vi "DDS RAM Set.vi"(8 "error in (no error)":errorcluster, 11 "DDS Box Cluster":T1 {"Array of DDS Channels (4)"."Channel Parameters"."Ref Clock Rate [kHz]" min=0.0}) -> (0 "error out":errorcluster, 3 "DDS box device reference":T2={"NI USB-8451 device reference"="", "DIO port"=0, "Serial Clock Rate [kHz]"=1000})   [LabVIEW 2013]
uses:
  DDS_box_device_reference.ctl
  <vilib>/ni845x/ni845x.llb/ni845xControl.ctl
  DDS_box_cluster.ctl
  array_of_DDS_channels.ctl
  DDS_channel.ctl
  array_of_DDS_profiles.ctl
  DDS_profile.ctl
  DDS RAM mode.ctl
  AD9910 registers.ctl
  <vilib>/gmath/NI_Gmath.lvlib
  cesium_controller/DDS/DDS.lvclass
panel:
  out "RAM data":u8[][](array[numeric])
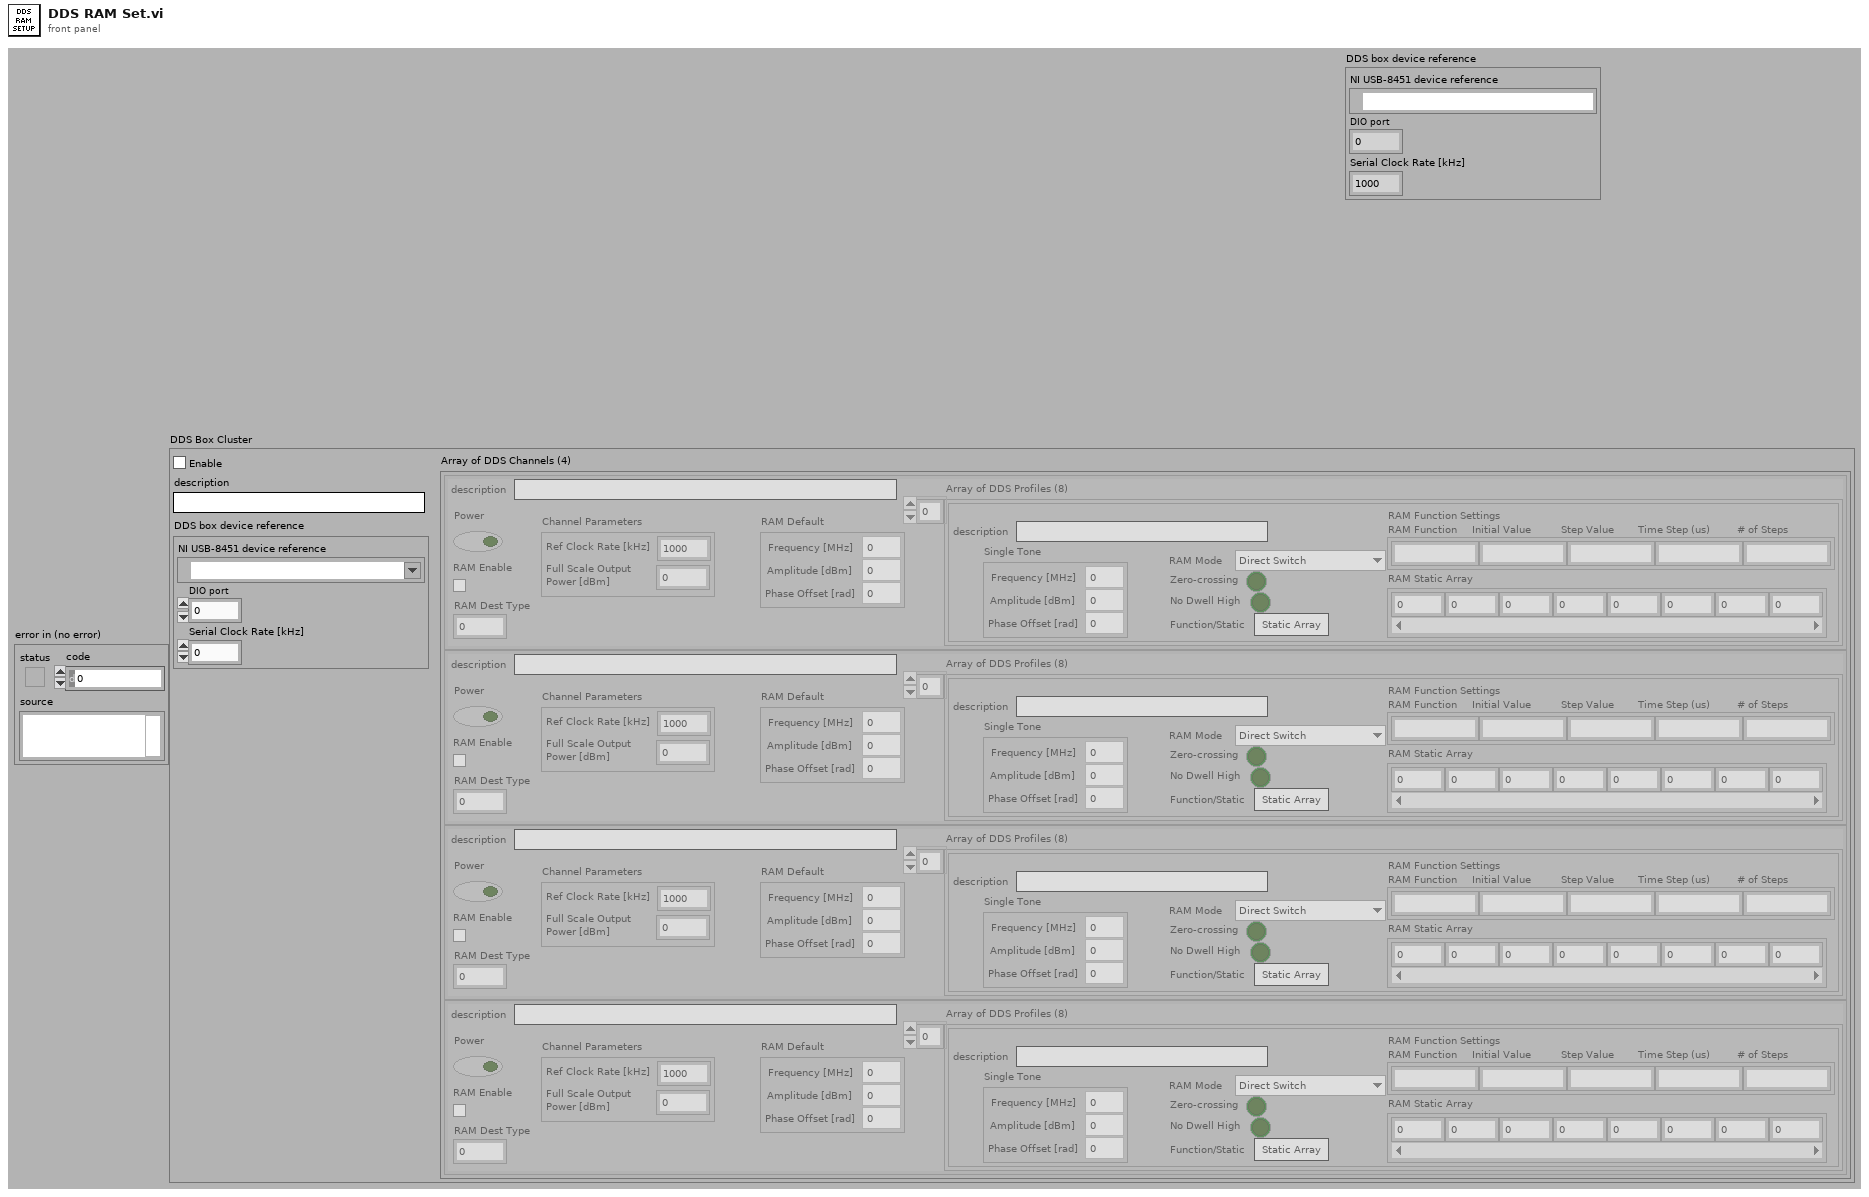
[diagram p1: front panel]
types:
  T1 = typedef "DDS_box_cluster.ctl" = cluster{"DDS box device reference":T2, "Array of DDS Channels (4)":T4, "Enable":bool, "description":string}
  T2 = typedef "DDS_box_device_reference.ctl" = cluster{"NI USB-8451 device reference":T3, "DIO port":u8, "Serial Clock Rate [kHz]":u16}
  T3 = typedef "ni845xControl.ctl" = refnum<k21>
  T4 = typedef "DDS.lvclass/array_of_DDS_channels.ctl" = T5[]
  T5 = typedef "DDS.lvclass/DDS_channel.ctl" = cluster{"Power":bool, "Channel Parameters":cluster{"Ref Clock Rate [kHz]":dbl, "Full Scale Output\nPower [dBm]":dbl}, "RAM Enable":bool, "RAM Dest Type":u8, "RAM Default":cluster{"Frequency [MHz]":dbl, "Amplitude [dBm]":dbl, "Phase Offset [rad]":dbl}, "Array of DDS Profiles (8)":T6, "description":string}
  T6 = typedef "DDS.lvclass/array_of_DDS_profiles.ctl" = T7[]
  T7 = typedef "DDS_profile.ctl" = cluster{"Single Tone":cluster{"Frequency [MHz]":dbl, "Amplitude [dBm]":dbl, "Phase Offset [rad]":dbl}, "RAM Mode ":T8, "Zero-crossing":bool, "No Dwell High":bool, "Function/Static":bool, "RAM Function Settings":string[], "RAM Static Array":dbl[], "description":string}
  T8 = typedef "DDS RAM mode.ctl" = enum16{"Direct Switch", "Ramp Up", "Bidirectional Ramp", "Continuous Bidirectional Ramp", "Continuous Recirculate", "Direct Switch 2", "Direct Switch 3", "Direct Switch 4"}
  T9 = typedef "AD9910 registers.ctl" = enum16{"CFR1", "CFR2", "CFR3", "Auxiliary DAC Control", "I/0 Update Rate", "Frequency Tuning Word", "Phase Offset Word", "Amplitude Scale Factor", "Multichip Sync", "Digital Ramp Limit", "Digital Ramp Step Size", "Digital Ramp Rate", "Single Tone Profile 0", "Single Tone Profile 1", "Single Tone Profile 2", "Single Tone Profile 3", "Single Tone Profile 4", "Single Tone Profile 5", "Single Tone Profile 6", "Single Tone Profile 7", "RAM Profile 0", "RAM Profile 1", "RAM Profile 2", "RAM Profile 3", "RAM Profile 4", "RAM Profile 5", "RAM Profile 6", "RAM Profile 7", "RAM"}
  T10 = cluster{"Ref Clock Rate [kHz]":dbl, "Full Scale Output\nPower [dBm]":dbl}
  T11 = cluster{"Frequency [MHz]":dbl, "Amplitude [dBm]":dbl, "Phase Offset [rad]":dbl}
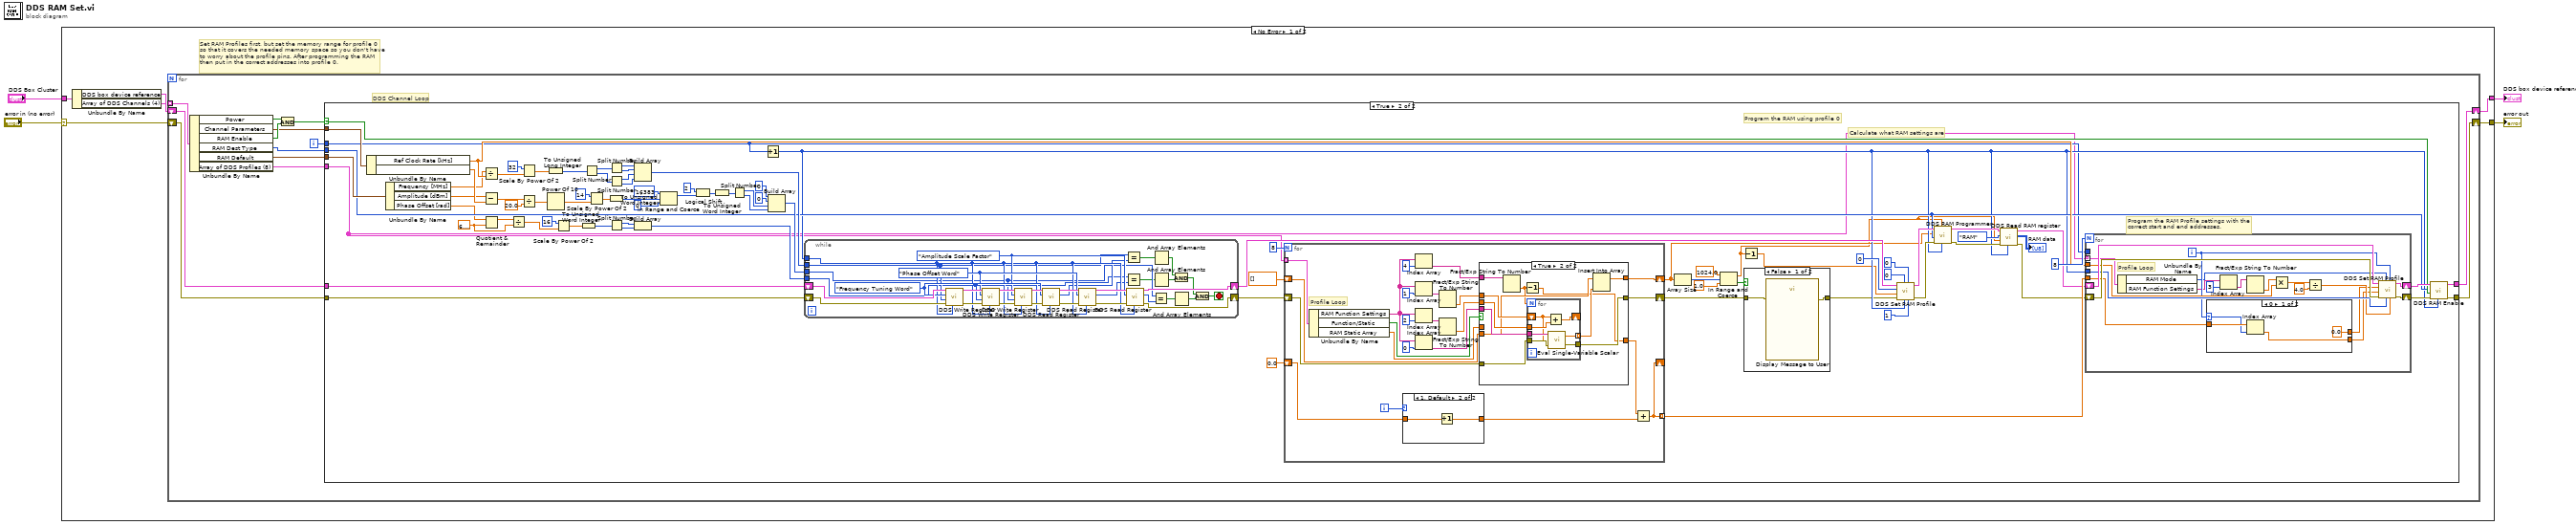
[diagram p0: block diagram]
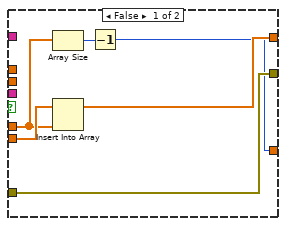
[diagram p5: hidden frame]
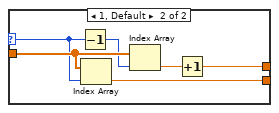
[diagram p6: hidden frame]
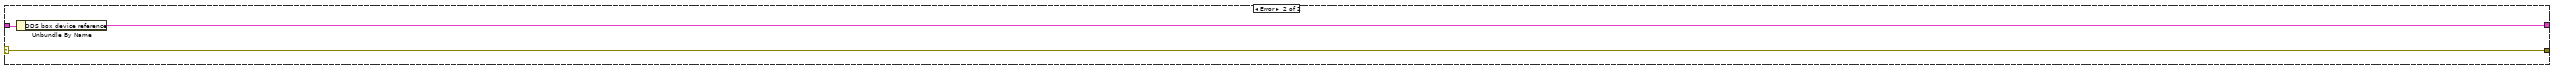
[diagram p7: hidden frame]
diagram:
  n1 = case shown="No Error" "error in (no error)" {
    selector: "error in (no error)" -> [w6 w225]
    tunnel: [w10 w226] -> w4
    tunnel: [w9 w225] -> w3
    tunnel: "DDS Box Cluster" -> [w5 w224]
    frame No Error {
      # "Set RAM Profiles first, but set the memory range for profile 0\nso that it covers the needed memory space so you don't have\nto worry about the profile pins. After programming the RAM\nthen put in the correct addresses into profile 0."
      n2 = Unbundle By Name(w5) -> ("DDS box device reference"=w8:T2, "Array of DDS Channels (4)"=w7:T4)
      n3 = for {
        shift-right: [w23] -> w10
        shift-left: w8 -> [w21]
        shift-right: [w22] -> w9
        shift-left: w6 -> [w20]
        tunnel: w7 -> [w18] mode=indexing
        i -> [w19]
        # "DDS Channel Loop"
        n4 = Unbundle By Name(w18) -> ("Power"=w17:bool, "Channel Parameters"=w14:T10, "RAM Enable"=w16:bool, "RAM Dest Type"=w13:u8, "RAM Default"=w12:T11, "Array of DDS Profiles (8)"=w11:T6)
        n5 = And(x=w17, y=w16) -> (x .and. y?=w15:bool)
        n6 = case shown="True" w15 {
          selector: w15 -> [_ w56]
          tunnel: w12 -> [_ w81]
          tunnel: w14 -> [_ w80]
          tunnel: [w25 w59] -> w23
          tunnel: [w24 w57] -> w22
          tunnel: w21 -> [w25 w61]
          tunnel: w20 -> [w24 w26]
          tunnel: w13 -> [_ w55]
          tunnel: w19 -> [_ w31]
          tunnel: w11 -> [_ w30]
          frame False {
          }
          frame True {
            w95 = 6.283185307179586
            # "Program the RAM Profile settings with the\ncorrect start and end addresses."
            # "Program the RAM using profile 0"
            # "Calculate what RAM settings are"
            n7 = Unbundle By Name(w80) -> ("Ref Clock Rate [kHz]"=w74:dbl, "Full Scale Output\nPower [dBm]"=w79:dbl)
            n8 = Unbundle By Name(w81) -> ("Frequency [MHz]"=w29:dbl, "Amplitude [dBm]"=w28:dbl, "Phase Offset [rad]"=w27:dbl)
            n9 = Divide(x=w29, y=w74) -> (x/y=w109:dbl)
            n10 = Subtract(x=w28, y=w79) -> (x-y=w91:dbl)
            n11 = Quotient & Remainder(x=w27, y=w95) -> (x-y*floor(x/y)=w98:dbl)  [unwired: 1 out]
            n12 = Divide(x=w98, y=w95) -> (x/y=w96:dbl)
            n13 = Scale By Power Of 2(n=32 ("x"), x=w109) -> (x*2^n=w107:dbl)
            n14 = Divide(x=w91, y=20.0) -> (x/y=w89:dbl)
            n15 = To Unsigned Long Integer(number=w107) -> (unsigned 32bit integer=w104:u32)
            n16 = Power Of 10(x=w89) -> (10^x=w88:dbl)
            n17 = Scale By Power Of 2(n=16, x=w96) -> (x*2^n=w97:dbl)
            n18 = To Unsigned Word Integer(number=w97) -> (unsigned 16bit integer=w94:u16)
            n19 = Split Number(x=w104) -> (hi(x)=w105:u16, lo(x)=w106:u16)
            n20 = Scale By Power Of 2(n=14, x=w88) -> (x*2^n=w86:dbl)
            n21 = To Unsigned Word Integer(number=w86) -> (unsigned 16bit integer=w51:u16)
            n22 = Split Number(x=w105) -> (hi(x)=w103:u8, lo(x)=w102:u8)
            n23 = Split Number(x=w106) -> (hi(x)=w101:u8, lo(x)=w100:u8)
            n24 = Split Number(x=w94) -> (hi(x)=w93:u8, lo(x)=w92:u8)
            n25 = Build Array(w103, w102, w101, w100) -> (w78:u8[])
            n26 = Build Array(w93, w92) -> (w76:u8[])
            n27 = In Range and Coerce(upper limit=u32 16383, x=w51, lower limit=u32 0) -> (coerced(x)=w50:u32)  [unwired: 1 out]
            n28 = Logical Shift(y=i8 2, x=w50) -> (x << y=w49:u32)
            n29 = To Unsigned Word Integer(number=w49) -> (unsigned 16bit integer=w48:u16)
            n30 = Split Number(x=w48) -> (hi(x)=w84:u8, lo(x)=w85:u8)
            n31 = Increment(x=w31) -> (x+1=w42:i32)
            n32 = Build Array(u8 0 ("element"), u8 0 ("element"), w84, w85) -> (w77:u8[])
            n33 = while {
              tunnel: w78 -> [w125]
              tunnel: w77 -> [w123]
              tunnel: w76 -> [w124]
              tunnel: w42 -> [w127]
              shift-right: [w131] -> w73
              shift-left: w61 -> [w140]
              shift-right: [w132] -> w71
              shift-left: w26 -> [w139]
              stop <- w113 stop-if-true
              w128 = AD9910_registers."Amplitude Scale Factor" ("Register")
              w129 = AD9910_registers."Phase Offset Word" ("Register")
              w130 = AD9910_registers."Frequency Tuning Word" ("Register")
              n34 = call "DDS Write Register.vi"("channel number (1)"=w127, "error in (no error)"=w139, "Write Data"=w125, "Register"=w130, "DDS ref in"=w140) -> ("error out"=w143:errorcluster, "DDS ref out"=w144:T2)  [unwired: 5 in]
              n35 = call "DDS Write Register.vi"("channel number (1)"=w127, "error in (no error)"=w143, "Write Data"=w124, "Register"=w129, "DDS ref in"=w144) -> ("error out"=w141:errorcluster, "DDS ref out"=w142:T2)  [unwired: 5 in]
              n36 = call "DDS Write Register.vi"("channel number (1)"=w127, "error in (no error)"=w141, "Write Data"=w123, "Register"=w128, "DDS ref in"=w142) -> ("error out"=w135:errorcluster, "DDS ref out"=w138:T2)  [unwired: 5 in]
              n37 = call "DDS Read Register.vi"("channel number (1)"=w127, "error in (no error)"=w135, "Register"=w130, "DDS ref in"=w138) -> ("error out"=w134:errorcluster, "Read data"=w126:u8[], "DDS ref out"=w137:T2)  [unwired: 5 in]
              n38 = call "DDS Read Register.vi"("channel number (1)"=w127, "error in (no error)"=w134, "Register"=w129, "DDS ref in"=w137) -> ("error out"=w133:errorcluster, "Read data"=w122:u8[], "DDS ref out"=w136:T2)  [unwired: 5 in]
              n39 = Equal?(x=w125, y=w126) -> (x = y?=w120:bool[])
              n40 = Equal?(x=w124, y=w122) -> (x = y?=w118:bool[])
              n41 = call "DDS Read Register.vi"("channel number (1)"=w127, "error in (no error)"=w133, "Register"=w128, "DDS ref in"=w136) -> ("error out"=w132:errorcluster, "Read data"=w121:u8[], "DDS ref out"=w131:T2)  [unwired: 5 in]
              n42 = And Array Elements(Boolean array=w120) -> (logical AND=w116:bool)
              n43 = And Array Elements(Boolean array=w118) -> (logical AND=w117:bool)
              n44 = Equal?(x=w123, y=w121) -> (x = y?=w119:bool[])
              n45 = And(x=w116, y=w117) -> (x .and. y?=w114:bool)
              n46 = And Array Elements(Boolean array=w119) -> (logical AND=w115:bool)
              n47 = And(x=w114, y=w115) -> (x .and. y?=w113:bool)
            }
            n48 = for {
              N: 8 -> [_]
              shift-right: [w166] -> w40
              shift-left: dbl[] [] -> [w167]
              shift-right: [w157] -> _
              shift-left: 0.0 -> [w159]
              shift-right: [w163] -> w33
              shift-left: w71 -> [w162]
              tunnel: [w157] -> w70 mode=indexing
              tunnel: w30 -> [w148] mode=indexing
              i -> [w160]
              # "Profile Loop"
              n49 = Unbundle By Name(w148) -> ("RAM Function Settings"=w146:string[], "Function/Static"=w145:bool, "RAM Static Array"=w147:dbl[])
              n50 = case shown="1, Default" w160 {
                tunnel: w159 -> [w168 w170]
                tunnel: [w168 w169] -> w158
                frame 0 {
                }
                frame 1, Default {
                  n51 = Increment(x=w170) -> (x+1=w169:dbl)
                }
              }
              n52 = Index Array(array=w146, index=4) -> (element=w149:string)
              n53 = Index Array(array=w146, index=1) -> (element=w151:string)
              n54 = Index Array(array=w146, index=2) -> (element=w150:string)
              n55 = Index Array(array=w146, index=0) -> (element=w152:string)
              n56 = Fract/Exp String To Number(string=w151) -> (number=w165:dbl)  [unwired: 3 in, 1 out]
              n57 = Fract/Exp String To Number(string=w150) -> (number=w164:dbl)  [unwired: 3 in, 1 out]
              n58 = case shown="True" w145 {
                tunnel: w152 -> [_ w187]
                tunnel: w165 -> [_ w185]
                tunnel: [w174 w183] -> w166
                tunnel: w164 -> [_ w186]
                tunnel: w167 -> [w175 w184]
                tunnel: [w172 w177] -> w161
                tunnel: [w176 w181] -> w163
                tunnel: w162 -> [w176 w180]
                tunnel: w147 -> [w171 _]
                tunnel: w149 -> [_ w179]
                frame False {
                  n59 = Array Size(array=w171) -> (size(s)=w173:i32)
                  n60 = Insert Into Array(array=w175, new element=w171) -> (w174:dbl[])  [unwired: 1 in]
                  n61 = Decrement(x=w173) -> (x-1=w172:i32)
                }
                frame True {
                  n62 = Fract/Exp String To Number(string=w179) -> (number=w178:dbl)  [unwired: 3 in, 1 out]
                  n63 = Decrement(x=w178) -> (x-1=w177:dbl)
                  n64 = for {
                    N: w178 -> [_]
                    tunnel: w187 -> [w194]
                    tunnel: [w193] -> w182 mode=indexing
                    tunnel: w186 -> [w192]
                    shift-right: [w191] -> _
                    shift-left: w185 -> [w188]
                    tunnel: [w190] -> w181
                    tunnel: w180 -> [w189]
                    n65 = Add(x=w188, y=w192) -> (x+y=w191:dbl)
                    n66 = call <vilib>:"Eval Single-Variable Scalar.vi"("error in (no error)"=w189, "x value"=w188, "formula"=w194) -> ("error out"=w190:errorcluster, "y value"=w193:dbl)
                  }
                  n67 = Insert Into Array(array=w184, new element=w182) -> (w183:dbl[])  [unwired: 1 in]
                }
              }
              n68 = Add(x=w161, y=w158) -> (x+y=w157:dbl)
            }
            n69 = Array Size(array=w40) -> (size(s)=w36:i32)
            n70 = In Range and Coerce(upper limit=1024.0, x=w36, lower limit=1.0) -> (coerced(x)=w35:dbl, In Range?=w34:bool)
            n71 = Decrement(x=w35) -> (x-1=w39:dbl)
            n72 = case shown="False" w34 {
              tunnel: w33 -> [w111 w112]
              tunnel: [w110 w112] -> w32
              frame False {
                n73 = call "Display Message to User"("error in (no error)"=w111) -> ("error out"=w110:errorcluster)  [unwired: 9 in, 1 out]
              }
              frame True {
              }
            }
            n74 = call "DDS Set RAM Profile.vi"("Step Rate"=u16 1, "Profile (0)"=u8 0, "channel number (1)"=w42, "RAM mode"=u8 0, "error in (no error)"=w32, "End Address"=w39, "Start Address"=u16 0, "DDS ref in"=w73) -> ("error out"=w66:errorcluster, "DDS ref out"=w67:T2)  [unwired: 1 in, 1 out]
            n75 = call "DDS RAM Programmer.vi"("channel number (1)"=w42, "# of Words"=w35, "error in (no error)"=w66, "RAM Destination"=w55, "RAM data"=w40, "DDS ref in"=w67) -> ("error out"=w46:errorcluster, "DDS ref out"=w47:T2)  [unwired: 3 in, 1 out]
            n76 = call "DDS Read RAM register.vi"("channel number (1)"=w42, "error in (no error)"=w46, "# of Words"=w35, "Register"=AD9910_registers."RAM", "DDS ref in"=w47) -> ("error out"=w45:errorcluster, "RAM data"=→"RAM data":u8[][], "DDS ref out"=w44:T2)  [unwired: 4 in]
            n77 = for {
              N: 8 -> [_]
              tunnel: w42 -> [w211]
              shift-right: [w209] -> w58
              shift-left: w45 -> [w212]
              shift-right: [w210] -> w60
              shift-left: w44 -> [w213]
              tunnel: w70 -> [w201]
              tunnel: w74 -> [w208]
              tunnel: w31 -> [_]
              tunnel: w30 -> [w197] mode=indexing
              i -> [w202]
              # "Profile Loop"
              n78 = Unbundle By Name(w197) -> ("RAM Mode"=w196:T8, "RAM Function Settings"=w199:string[])
              n79 = case shown="0" w202 {
                selector: w202 -> [w215 w222]
                tunnel: [0.0 w219] -> w203
                tunnel: w201 -> [w216 w223]
                tunnel: [w214 w218] -> w200
                frame 0 {
                  n80 = Index Array(array=w216, index=w215) -> (element=w214:dbl)
                }
                frame 1, Default {
                  n81 = Decrement(x=w222) -> (x-1=w221:i32)
                  n82 = Index Array(array=w223, index=w222) -> (element=w218:dbl)
                  n83 = Index Array(array=w223, index=w221) -> (element=w220:dbl)
                  n84 = Increment(x=w220) -> (x+1=w219:dbl)
                }
              }
              n85 = Index Array(array=w199, index=3) -> (element=w198:string)
              n86 = Fract/Exp String To Number(string=w198) -> (number=w204:dbl)  [unwired: 3 in, 1 out]
              n87 = Multiply(x=w204, y=w208) -> (x*y=w207:dbl)
              n88 = Divide(x=w207, y=4.0) -> (x/y=w205:dbl)
              n89 = call "DDS Set RAM Profile.vi"("Step Rate"=w205, "Profile (0)"=w202, "channel number (1)"=w211, "RAM mode"=w196, "error in (no error)"=w212, "End Address"=w200, "Start Address"=w203, "DDS ref in"=w213) -> ("error out"=w209:errorcluster, "DDS ref out"=w210:T2)  [unwired: 1 in, 1 out]
            }
            n90 = call "DDS RAM Enable.vi"("channel number (1)"=w42, "error in"=w58, "RAM Enable"=w56, "RAM Dest Type"=w55, "DDS ref in"=w60) -> ("error out"=w57:errorcluster, "DDS ref out"=w59:T2)  [unwired: 5 in]
          }
        }
      }
    }
    frame Error {
      n91 = Unbundle By Name(w224) -> ("DDS box device reference"=w226:T2)
    }
  }
  "error out" <- w3
  "DDS box device reference" <- w4
